vi "RSZVB Get TRM Pulse Generator Source.vi"(8 "error in (no error)":errorcluster {"code" format="%.0x"}, 9 "Ext Out (1)":i32=1, 10 "Channel (1)":i32=1, 11 "VISA resource name":refnum<visa-resource-name>) -> (0 "error out":errorcluster {"code" format="%.0x"}, 2 "Pulse Generator Source":i32, 3 "VISA resource name out":refnum<visa-resource-name>)   [LabVIEW 2011]
doc: "This VI returns the source signal for pulse generator output <No> of the R&S ZVAX-TRM.\n\nRemote-control command(s):\n[SENSe<Ch>:]TEUNit:REAR<No>:SOURce?"
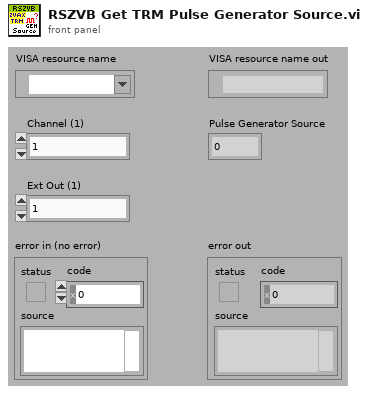
[diagram p1: front panel]
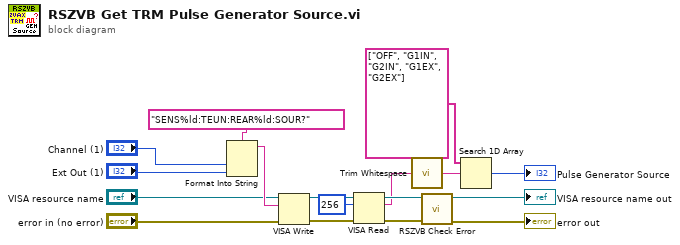
[diagram p0: block diagram]
diagram:
  n1 = Format Into String(format string="SENS%ld:TEUN:REAR%ld:SOUR?", "Channel (1)", "Ext Out (1)") -> (resulting string=w17:string)  [unwired: 2 in, 1 out]
  n2 = VISA Write(VISA resource name="VISA resource name", write buffer=w17, error in (no error)="error in (no error)") -> (VISA resource name out=w15:refnum<visa-resource-name>, error out=w14:errorcluster)  [unwired: 1 out]
  n3 = VISA Read(VISA resource name=w15, byte count=u32 256, error in (no error)=w14) -> (VISA resource name out=w12:refnum<visa-resource-name>, read buffer=w11:string, error out=w13:errorcluster)  [unwired: 1 out]
  n4 = call <vilib>:"Trim Whitespace.vi"("string"=w11) -> ("trimmed string"=w10:string)  [unwired: 1 in]
  n5 = call "RSZVB Check Error.vi"("error in (no error)"=w13, "VISA session"=w12) -> ("error out"=→"error out":errorcluster, "dup VISA session"=→"VISA resource name out":refnum<visa-resource-name>)  [unwired: 8 in]
  n6 = Search 1D Array(1D array=string[] ["OFF", "G1IN", "G2IN", "G1EX", "G2EX"], element=w10) -> (index of element=→"Pulse Generator Source":i32)  [unwired: 1 in]
